vi "AVI-Write.vi"() -> (0 "ErrOut":errorcluster)   [LabVIEW 2014]
doc: "Use this template to build a VI to use as a subVI."
uses:
  <vilib>/vision/NI_Vision_Development_Module.lvlib
panel:
  in  "ErrIn":errorcluster
  # "Input Parameters"
  # "Output Parameters"
  # "VI Description:\nThis VI is .."
  # ":: MVI Framework V1.0 ::\nAuthor:Gaoke Yang\nEmail: gaoke.yang@yahoo.com\nWeb: www.mvicontrol.com\nCopyright (C) 2014, MVI Technologies All Rights Reserved"
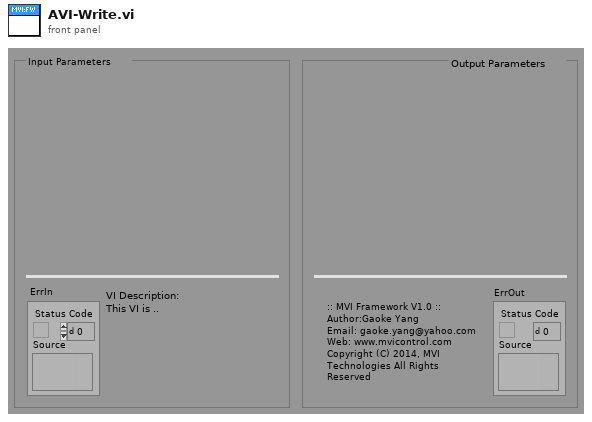
[diagram p1: front panel]
types:
  T1 = typedef "Image Type" = u32
  T2 = typedef "IMAQ Image.ctl" = refnum<image>
  T3 = typedef "IMAQ AVI2 Refnum.ctl" = refnum<k20>
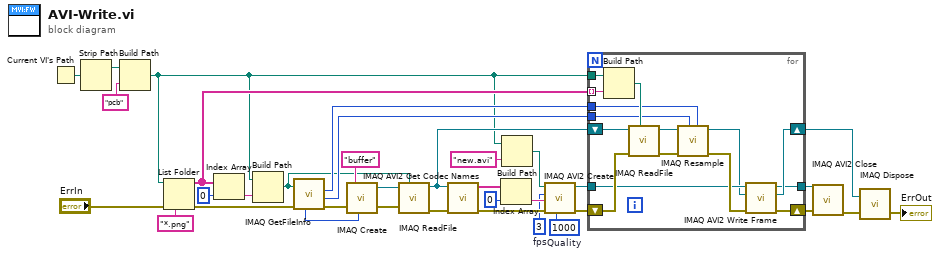
[diagram p0: block diagram]
diagram:
  w1 = 1000  # Quality
  w2 = u32 3  # fps
  n1 = Current VI's Path() -> (path=w13:path)
  n2 = Strip Path(path=w13) -> (stripped path=w12:path)  [unwired: 1 out]
  n3 = Build Path(base path=w12, name or relative path="pcb") -> (appended path=w4:path)
  n4 = List Folder(path=w4, pattern="*.png", error in="ErrIn") -> (filenames=w20:string[], error out=w10:errorcluster)  [unwired: 3 out]
  n5 = Index Array(array=w20, index=0) -> (element=w28:string)
  n6 = Build Path(base path=w4, name or relative path=w28) -> (appended path=w6:path)
  n7 = call "IMAQ GetFileInfo"("error in (no error)"=w10, "File Path"=w6) -> ("error out"=w8:errorcluster, "Y Resolution"=w26:i32, "X Resolution"=w27:i32, "Image Type"=w11:T1)  [unwired: 3 in, 3 out]
  n8 = call "IMAQ Create"("Image Name"="buffer", "Image Type"=w11, "error in (no error)"=w8) -> ("New Image"=w30:T2, "error out"=w9:errorcluster)  [unwired: 1 in, 1 out]
  n9 = call "IMAQ ReadFile"("File Path"=w6, "error in (no error)"=w9, "Image"=w30) -> ("error out"=w7:errorcluster, "Image Out"=w19:T2)  [unwired: 2 in, 5 out]
  n10 = call "IMAQ AVI2 Get Codec Names"("error in (no error)"=w7, "Image"=w19) -> ("error out"=w31:errorcluster, "Codec Names"=w23:string[])  [unwired: 8 in]
  n11 = Index Array(array=w23, index=0) -> (element=w24:string)
  n12 = Build Path(base path=w4, name or relative path="new.avi") -> (appended path=w34:path)
  n13 = call "IMAQ AVI2 Create"("Quality"=w1, "error in (no error)"=w31, "Codec"=w24, "Frames Per Second"=w2, "AVI Path"=w34) -> ("error out"=w21:errorcluster, "AVI Refnum"=w22:T3)  [unwired: 5 in]
  n14 = for {
    tunnel: w20 -> [w49] mode=indexing
    tunnel: w27 -> [w43]
    tunnel: w26 -> [w42]
    tunnel: w22 -> [w40]
    shift-right: [w39] -> w18
    shift-left: w21 -> [w46]
    shift-right: [w37] -> w16
    shift-left: w19 -> [w47]
    tunnel: w4 -> [w50]
    tunnel: [w36] -> w17
    n15 = Build Path(base path=w50, name or relative path=w49) -> (appended path=w48:path)
    n16 = call "IMAQ ReadFile"("File Path"=w48, "error in (no error)"=w46, "Image"=w47) -> ("error out"=w44:errorcluster, "Image Out"=w45:T2)  [unwired: 2 in, 5 out]
    n17 = call "IMAQ Resample"("X Resolution"=w43, "Y Resolution"=w42, "error in (no error)"=w44, "Image Src"=w45) -> ("error out"=w41:errorcluster, "Image Dst Out"=w38:T2)  [unwired: 6 in]
    n18 = call "IMAQ AVI2 Write Frame"("error in (no error)"=w41, "Image"=w38, "AVI Refnum"=w40) -> ("error out"=w39:errorcluster, "Image Out (duplicate)"=w37:T2, "AVI Refnum (duplicate)"=w36:T3)  [unwired: 6 in]
  }
  n19 = call "IMAQ AVI2 Close"("error in (no error)"=w18, "AVI Refnum"=w17) -> ("error out"=w15:errorcluster)  [unwired: 9 in]
  n20 = call "IMAQ Dispose"("Image"=w16, "error in (no error)"=w15) -> ("error out"=→"ErrOut":errorcluster)  [unwired: 4 in]
